vi "SetArmSetpoint.vi"(11 "Buttons":bool[](array[boolean])) -> ()   [LabVIEW 2014]
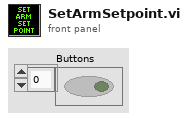
[diagram p1: front panel]
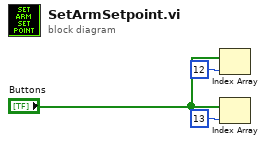
[diagram p0: block diagram]
diagram:
  n1 = Index Array(array="Buttons", index=12) -> ()  [unwired: 1 out]
  n2 = Index Array(array="Buttons", index=13) -> ()  [unwired: 1 out]
